vi "load_automatic_steps.vi"(8 "error in (no error)":errorcluster) -> (0 "error out":errorcluster, 2 "replaced_step(s)":bool, 3 "automatic_steps out":variant)   [LabVIEW 2015, in "example_01.lvlib"]
uses:
  example_01.lvlib
  lv-recipe-machine/public/_controls/step.ctl
  _controls/automatic_steps.ctl
  lv-recipe-machine/public/_controls/vi_reference_type.ctl
  automatic_steps/automatic_test_random.vi
  automatic_steps/automatic_test_comparison.vi
  automatic_steps/automatic_wait.vi
  automatic_steps/automatic_complete_continue.vi
  automatic_steps/automatic_complete_fail.vi
  automatic_steps/automatic_complete_finish.vi
  automatic_steps/automatic_transition.vi
  lv-recipe-machine/lv-recipe-machine.lvlib
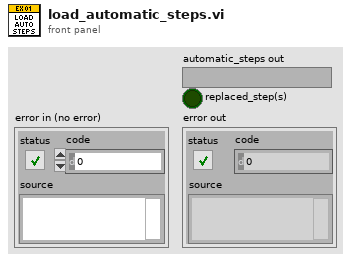
[diagram p1: front panel]
types:
  T1 = typedef "example_01.lvlib/automatic_steps.ctl" = enum16{"<automatic_step>", "auto_initialize", "auto_test_random", "auto_test_comparison", "auto_wait", "auto_complete_continue", "auto_complete_fail", "auto_complete_finish", "auto_transition", "<null>"}
  T2 = typedef "lv-recipe-machine.lvlib/vi_reference_type.ctl" = enum16{"<vi_reference_type>", "manual_action", "auto_step", "auto_criteria", "auto_transition", "<null>"}
  T3 = typedef "lv-recipe-machine.lvlib/step.ctl" = cluster{"name":string, "data":variant, "vi_reference":variant}
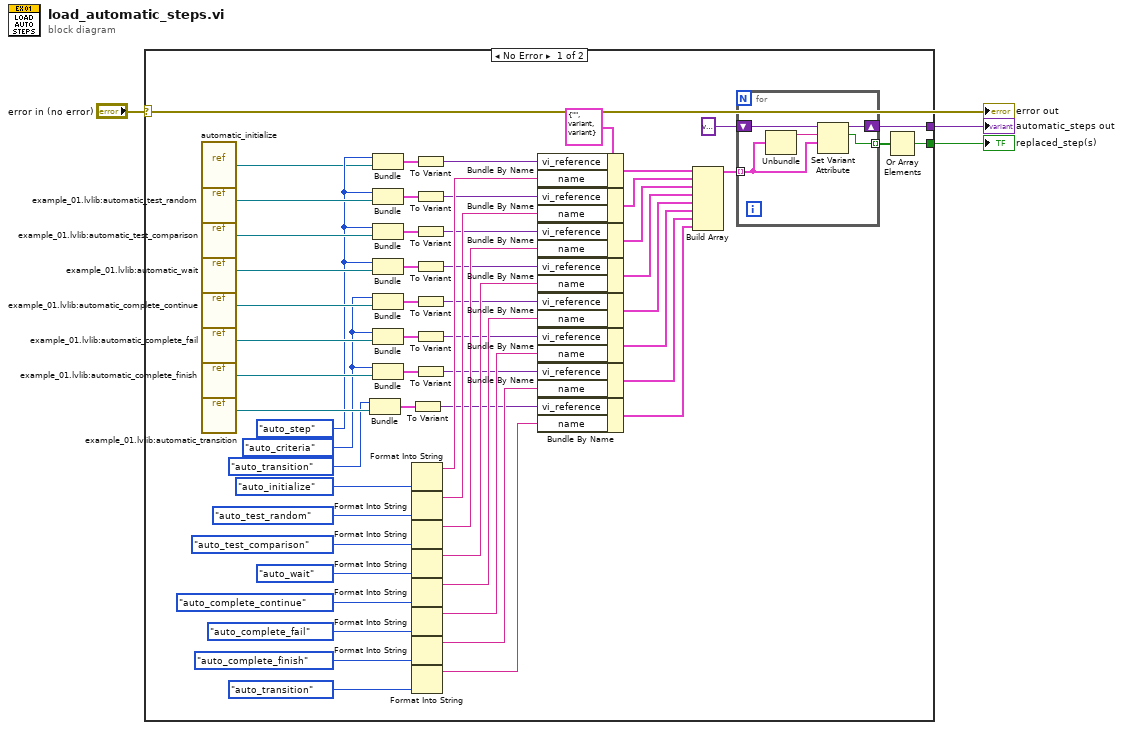
[diagram p0: block diagram]
diagram:
  n1 = case shown="No Error" "error in (no error)" {
    tunnel: [w55 _] -> w3
    tunnel: [w50 _] -> w2
    frame No Error {
      w12 = vi_reference_type."auto_criteria" ("vi_reference_type")
      w13 = vi_reference_type."auto_step" ("vi_reference_type")
      w9 = T3 {"name"="", "data"=variant, "vi_reference"=variant(refnum<vi> refnum)} ("step")
      n2 = vi-ref "automatic_initialize.vi"() -> (w4:refnum<vi>)
      n3 = vi-ref "example_01.lvlib:automatic_test_random.vi"() -> (w33:refnum<vi>)
      n4 = vi-ref "example_01.lvlib:automatic_test_comparison.vi"() -> (w32:refnum<vi>)
      n5 = vi-ref "example_01.lvlib:automatic_wait.vi"() -> (w31:refnum<vi>)
      n6 = vi-ref "example_01.lvlib:automatic_complete_continue.vi"() -> (w30:refnum<vi>)
      n7 = vi-ref "example_01.lvlib:automatic_complete_fail.vi"() -> (w29:refnum<vi>)
      n8 = vi-ref "example_01.lvlib:automatic_complete_finish.vi"() -> (w28:refnum<vi>)
      n9 = vi-ref "example_01.lvlib:automatic_transition.vi"() -> (w60:refnum<vi>)
      n10 = Bundle("vi_reference_type"=vi_reference_type."auto_transition", w60) -> (w7:cluster{"vi_reference_type":T2, refnum<vi>})  [unwired: 1 in]
      n11 = Bundle("vi_reference_type"=w13, w4) -> (w20:cluster{"vi_reference_type":T2, refnum<vi>})  [unwired: 1 in]
      n12 = Bundle("vi_reference_type"=w13, w33) -> (w19:cluster{"vi_reference_type":T2, refnum<vi>})  [unwired: 1 in]
      n13 = Bundle("vi_reference_type"=w13, w32) -> (w18:cluster{"vi_reference_type":T2, refnum<vi>})  [unwired: 1 in]
      n14 = Bundle("vi_reference_type"=w13, w31) -> (w17:cluster{"vi_reference_type":T2, refnum<vi>})  [unwired: 1 in]
      n15 = Bundle("vi_reference_type"=w12, w30) -> (w16:cluster{"vi_reference_type":T2, refnum<vi>})  [unwired: 1 in]
      n16 = Bundle("vi_reference_type"=w12, w29) -> (w15:cluster{"vi_reference_type":T2, refnum<vi>})  [unwired: 1 in]
      n17 = Bundle("vi_reference_type"=w12, w28) -> (w14:cluster{"vi_reference_type":T2, refnum<vi>})  [unwired: 1 in]
      n18 = Format Into String(automatic_steps."auto_initialize" ("automatic_steps")) -> (resulting string=w59:string)  [unwired: 3 in, 1 out]
      n19 = Format Into String(automatic_steps."auto_test_random" ("automatic_steps")) -> (resulting string=w58:string)  [unwired: 3 in, 1 out]
      n20 = Format Into String(automatic_steps."auto_test_comparison" ("automatic_steps")) -> (resulting string=w57:string)  [unwired: 3 in, 1 out]
      n21 = Format Into String(automatic_steps."auto_wait" ("automatic_steps")) -> (resulting string=w37:string)  [unwired: 3 in, 1 out]
      n22 = Format Into String(automatic_steps."auto_complete_continue" ("automatic_steps")) -> (resulting string=w36:string)  [unwired: 3 in, 1 out]
      n23 = Format Into String(automatic_steps."auto_complete_fail" ("automatic_steps")) -> (resulting string=w35:string)  [unwired: 3 in, 1 out]
      n24 = Format Into String(automatic_steps."auto_complete_finish" ("automatic_steps")) -> (resulting string=w34:string)  [unwired: 3 in, 1 out]
      n25 = Format Into String(automatic_steps."auto_transition" ("automatic_steps")) -> (resulting string=w8:string)  [unwired: 3 in, 1 out]
      n26 = To Variant(anything=w7) -> (Variant=w6:variant)
      n27 = To Variant(anything=w20) -> (Variant=w27:variant)
      n28 = To Variant(anything=w19) -> (Variant=w26:variant)
      n29 = To Variant(anything=w18) -> (Variant=w25:variant)
      n30 = To Variant(anything=w17) -> (Variant=w24:variant)
      n31 = To Variant(anything=w16) -> (Variant=w23:variant)
      n32 = To Variant(anything=w15) -> (Variant=w22:variant)
      n33 = To Variant(anything=w14) -> (Variant=w21:variant)
      n34 = Bundle By Name(cluster=w9, "vi_reference"=w27, "name"=w59) -> (w52:T3)
      n35 = Bundle By Name(cluster=w9, "vi_reference"=w26, "name"=w58) -> (w53:T3)
      n36 = Bundle By Name(cluster=w9, "vi_reference"=w25, "name"=w57) -> (w56:T3)
      n37 = Bundle By Name(cluster=w9, "vi_reference"=w24, "name"=w37) -> (w41:T3)
      n38 = Bundle By Name(cluster=w9, "vi_reference"=w23, "name"=w36) -> (w40:T3)
      n39 = Bundle By Name(cluster=w9, "vi_reference"=w22, "name"=w35) -> (w39:T3)
      n40 = Bundle By Name(cluster=w9, "vi_reference"=w21, "name"=w34) -> (w38:T3)
      n41 = Bundle By Name(cluster=w9, "vi_reference"=w6, "name"=w8) -> (w10:T3)
      n42 = Build Array(w52, w53, w56, w41, w40, w39, w38, w10) -> (w54:T3[])
      n43 = for {
        tunnel: w54 -> [w63] mode=indexing
        shift-right: [w64] -> w55
        shift-left: variant ("automatic_steps in") -> [w65]
        tunnel: [w61] -> w49 mode=indexing
        n44 = Unbundle(w63) -> ("name"=w62:string)  [unwired: 2 out]
        n45 = Set Variant Attribute(Variant=w65, name=w62, value=w63) -> (Variant out=w64:variant, replaced=w61:bool)  [unwired: 1 in, 1 out]
      }
      n46 = Or Array Elements(Boolean array=w49) -> (logical OR=w50:bool)
    }
    frame Error {
    }
  }
  "automatic_steps out" <- w3
  "replaced_step(s)" <- w2
  "error out" <- "error in (no error)"
